vi "Value_Occurence_Analysis.vi"(3 "Average Numeric Values?":bool, 4 "Tolerance":dbl=1.0 format="%.2f", 5 "Precision (3)":string, 6 "String Array":string[](array[string])) -> (0 "Numeric Array?":bool, 1 "St Dev":string, 2 "Output String":string)   [LabVIEW 2010]
uses:
  <vilib>/Analysis/NI_AALBase.lvlib
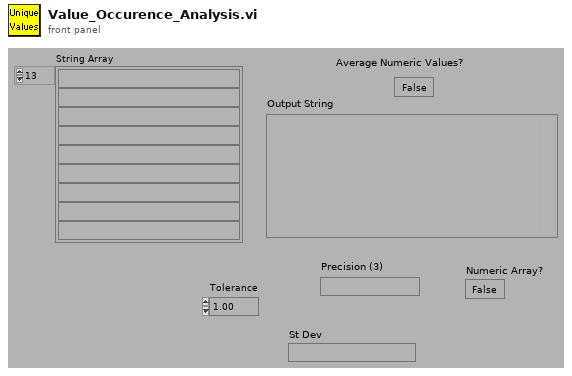
[diagram p1: front panel]
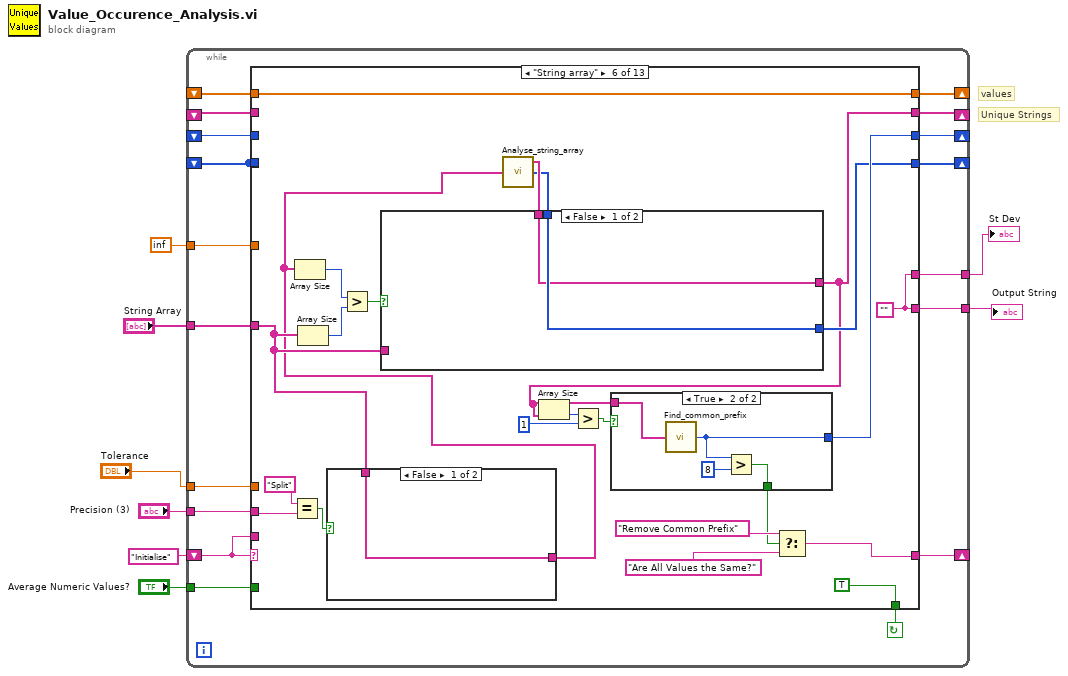
[diagram p0: block diagram]
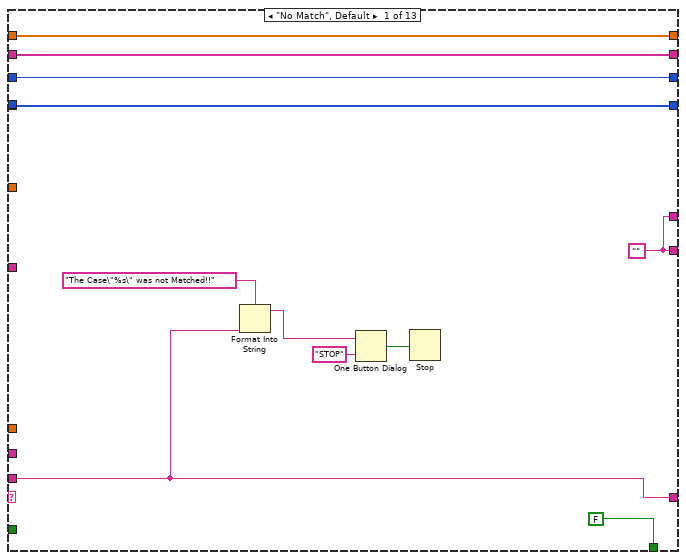
[diagram p2: hidden frame]
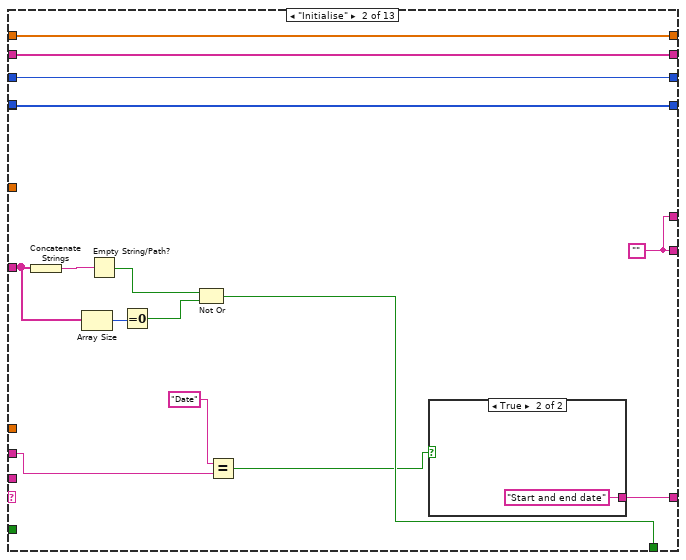
[diagram p3: hidden frame]
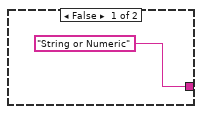
[diagram p4: hidden frame]
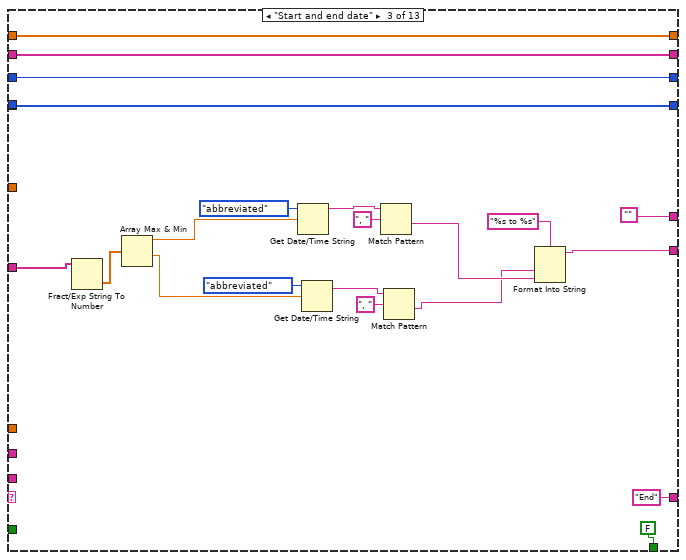
[diagram p5: hidden frame]
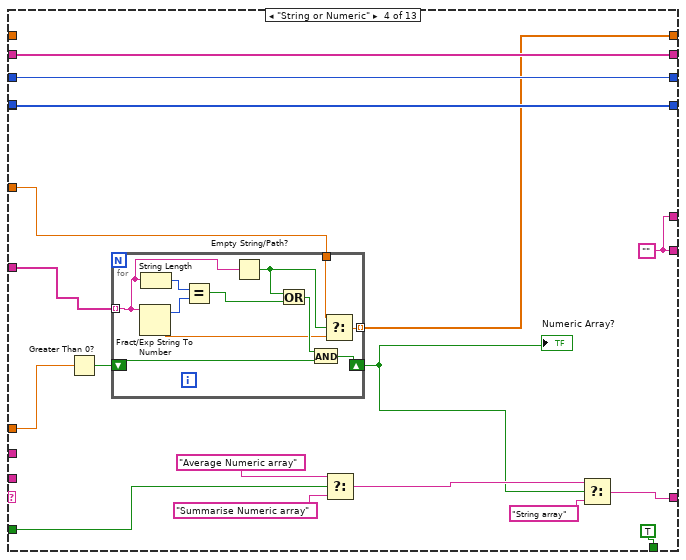
[diagram p6: hidden frame]
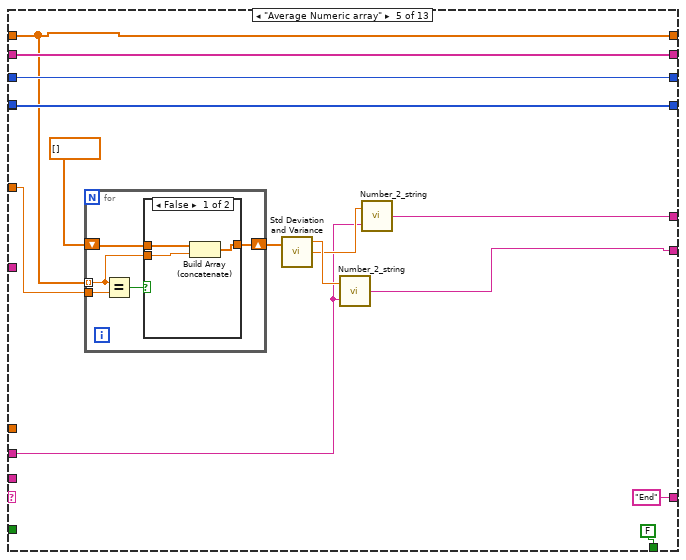
[diagram p7: hidden frame]
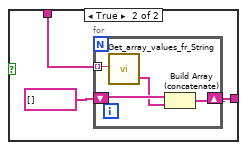
[diagram p9: hidden frame]
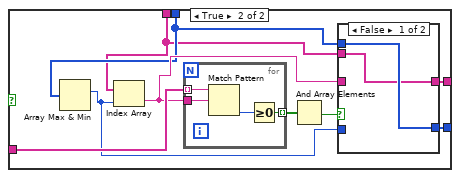
[diagram p10: hidden frame]
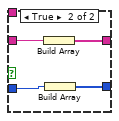
[diagram p11: hidden frame]
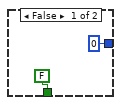
[diagram p12: hidden frame]
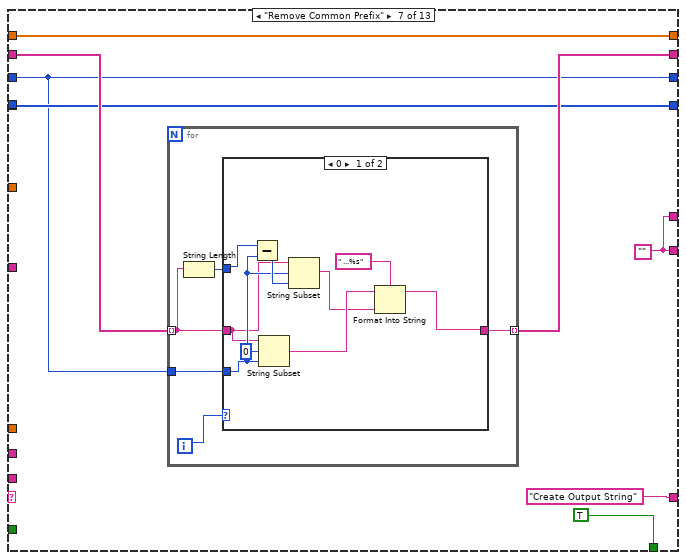
[diagram p13: hidden frame]
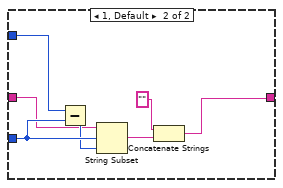
[diagram p14: hidden frame]
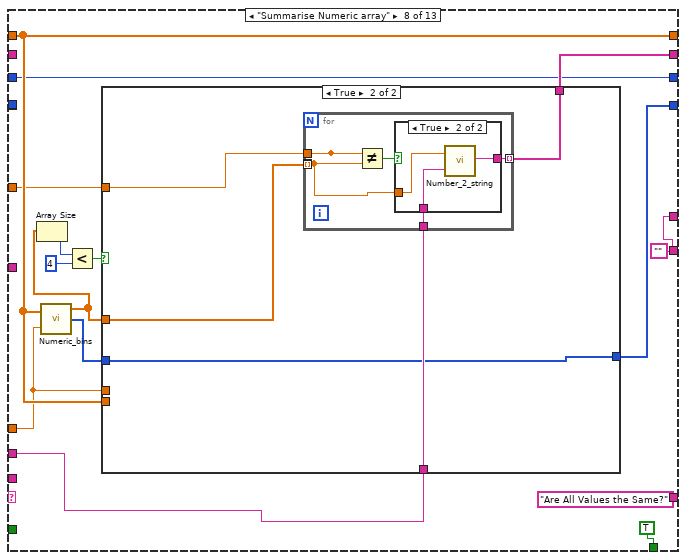
[diagram p15: hidden frame]
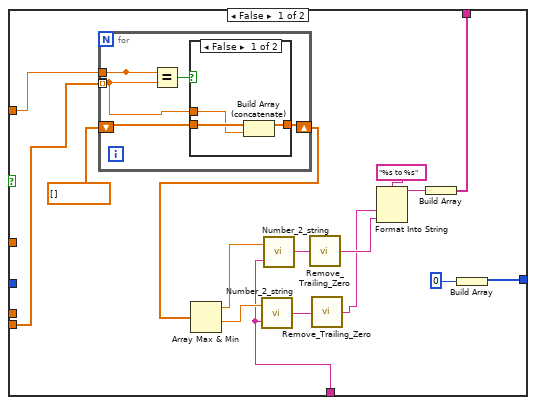
[diagram p16: hidden frame]
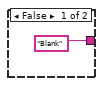
[diagram p18: hidden frame]
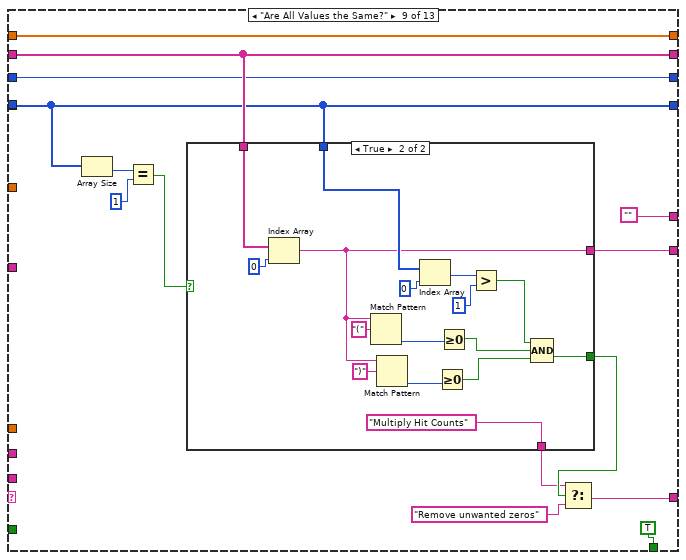
[diagram p19: hidden frame]
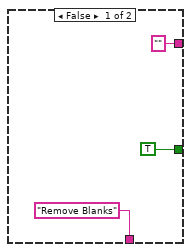
[diagram p20: hidden frame]
diagram:
  # "Unique Strings"
  # "values"
  n1 = while {
    shift-left: _ -> [w12]
    shift-right: [w13] -> _
    tunnel: [w14] -> w6
    shift-left: _ -> [w15]
    shift-right: [w16] -> _
    shift-left: _ -> [w17]
    shift-right: [w18] -> _
    tunnel: "Tolerance" -> [w19]
    shift-left: _ -> [w20]
    shift-right: [w24] -> _
    shift-left: "Initialise" -> [w21]
    shift-right: [w23] -> _
    tunnel: inf -> [w25]
    tunnel: "String Array" -> [w26]
    tunnel: "Average Numeric Values?" -> [w11]
    tunnel: "Precision (3)" -> [w10]
    tunnel: [w9] -> w2
    stop <- w22 continue-if-true
    n2 = case shown="\"String array\"" w21 {
      tunnel: w26 -> [_ w47 w62 w88 _ w135 _ _ _ _ _ _ _]
      tunnel: w25 -> [_ _ _ w76 w111 _ _ w223 _ _ _ _ _]
      tunnel: [w32 w52 w71 w77 w110 w148 w191 w225 w281 w313 w345 w378 w396] -> w24
      tunnel: [w33 w49 "End" w91 "End" w143 "Create Output String" "Are All Values the Same?" w269 "End" "Remove unwanted zeros" "Create Output String" "Initialise"] -> w23
      tunnel: [FALSE w43 FALSE TRUE FALSE TRUE TRUE TRUE TRUE FALSE TRUE TRUE FALSE] -> w22
      tunnel: w21 -> [w33 _ _ _ _ _ _ _ _ _ _ _ _]
      tunnel: w20 -> [w32 w52 w71 _ w110 w148 w191 w225 w281 w313 w345 w378 w396]
      tunnel: w19 -> [_ _ _ w86 _ _ _ w224 _ _ _ _ _]
      tunnel: [w30 w51 w73 w89 w116 w132 w187 w222 w274 w310 w342 w377 w386] -> w18
      tunnel: w17 -> [w30 w51 w73 w89 w116 _ w187 _ w274 w310 w344 w377 w386]
      tunnel: w17 -> [_ _ _ _ _ _ _ _ _ _ _ _ _]
      tunnel: [w29 w50 w75 w90 w117 w131 w189 w226 w278 w312 w343 w374 w393] -> w16
      tunnel: w15 -> [w29 w50 w75 w90 w117 _ w188 _ w278 w312 w341 w375 w393]
      tunnel: [w27 w41 w65 w78 w112 w139 w185 w214 w276 w304 w339 w373 w392] -> w14
      tunnel: [w28 w42 w74 w84 w114 w147 w186 w217 w277 w311 w340 w376 w391] -> w13
      tunnel: w12 -> [w28 w42 w74 w84 w114 _ w186 w217 w277 w311 w340 w376 w391]
      tunnel: w11 -> [_ _ _ w83 _ _ _ _ _ _ _ _ _]
      tunnel: w10 -> [_ w40 _ _ w105 w130 _ w215 _ _ _ _ _]
      tunnel: [w27 w41 "" w78 w104 w139 w185 w214 "" "" w339 w373 ""] -> w9
      frame "No Match", Default {
        w27 = ""
        n3 = Format Into String(format string="The Case\"%s\" was not Matched!!" ("Format String"), w33) -> (resulting string=w36:string)  [unwired: 2 in, 1 out]
        n4 = One Button Dialog(message=w36, button name ("OK")="STOP") -> (true=w31:bool)
        n5 = Stop(stop? (T)=w31) -> ()
      }
      frame "Initialise" {
        w41 = ""
        n6 = Concatenate Strings(w47) -> (w48:string)
        n7 = Array Size(array=w47) -> (size(s)=w45:i32)
        n8 = Empty String/Path?(string/path=w48) -> (empty?=w46:bool)
        n9 = Equal To 0?(x=w45) -> (x = 0?=w44:bool)
        n10 = Not Or(1:w44, 2:w46) -> (0:w43:bool)
        n11 = Equal?(x="Date", y=w40) -> (x = y?=w38:bool)
        n12 = case shown="True" w38 {
          tunnel: ["String or Numeric" "Start and end date"] -> w49
          frame False {
          }
          frame True {
          }
        }
      }
      frame "Start and end date" {
        n13 = Fract/Exp String To Number(string=w62) -> (number=w61:dbl[])  [unwired: 4 out]
        n14 = Array Max & Min(array=w61) -> (max value=w70:dbl, min value=w67:dbl)  [unwired: 2 out]
        n15 = Get Date/Time String(date format (0)=enum16{"short", "long", "abbreviated"}."abbreviated", seconds (now)=w70) -> (date string=w59:string)  [unwired: 2 out]
        n16 = Get Date/Time String(date format (0)=enum16{"short", "long", "abbreviated"}."abbreviated", seconds (now)=w67) -> (date string=w57:string)  [unwired: 2 out]
        n17 = Match Pattern(string=w59, regular expression=", ") -> (after substring=w56:string)  [unwired: 4 out]
        n18 = Match Pattern(string=w57, regular expression=", ") -> (after substring=w55:string)  [unwired: 4 out]
        n19 = Format Into String(format string="%s to %s", w55, w56) -> (resulting string=w65:string)  [unwired: 2 in, 1 out]
      }
      frame "String or Numeric" {
        w78 = ""
        n20 = Greater Than 0?(x=w86) -> (x > 0?=w85:bool)
        n21 = for {
          tunnel: w88 -> [w94] mode=indexing
          shift-right: [w101] -> w79
          shift-left: w85 -> [w102]
          tunnel: [w98] -> w77 mode=indexing
          tunnel: w76 -> [w99]
          n22 = Fract/Exp String To Number(string=w94) -> (offset past number=w96:i32, number=w97:dbl)  [unwired: 3 out]
          n23 = String Length(string=w94) -> (length=w95:i32)
          n24 = Equal?(x=w95, y=w96) -> (x = y?=w93:bool)
          n25 = Empty String/Path?(string/path=w94) -> (empty?=w100:bool)
          n26 = Or(x=w100, y=w93) -> (x .or. y?=w103:bool)
          n27 = And(x=w103, y=w102) -> (x .and. y?=w101:bool)
          n28 = Select(t=w99, s=w100, f=w97) -> (s? t:f=w98:dbl)
        }
        "Numeric Array?" <- w79
        n29 = Select(t="Average Numeric array", s=w83, f="Summarise Numeric array") -> (s? t:f=w80:string)
        n30 = Select(t=w80, s=w79, f="String array") -> (s? t:f=w91:string)
      }
      frame "Average Numeric array" {
        n31 = for {
          shift-right: [w118] -> w108
          shift-left: dbl[] [] -> [w120]
          tunnel: w111 -> [w122]
          tunnel: w110 -> [w119] mode=indexing
          n32 = Equal?(x=w119, y=w122) -> (x = y?=w121:bool)
          n33 = case shown="False" w121 {
            tunnel: w120 -> [w125 w126]
            tunnel: w119 -> [w124 _]
            tunnel: [w123 w126] -> w118
            frame False {
              n34 = Build Array (concatenate)(w125, w124) -> (w123:dbl[])
            }
            frame True {
            }
          }
        }
        n35 = call <vilib>:"Std Deviation and Variance.vi"("X"=w108) -> ("mean"=w107:dbl, "standard deviation"=w106:dbl)  [unwired: 1 in, 1 out]
        n36 = call "Number_2_string.vi"("precision"=w105, "number"=w107) -> ("String"=w112:string)
        n37 = call "Number_2_string.vi"("precision"=w105, "number"=w106) -> ("String"=w104:string)
      }
      frame "String array" {
        w139 = ""
        n38 = Equal?(x="Split", y=w130) -> (x = y?=w127:bool)
        n39 = Array Size(array=w135) -> (size(s)=w137:i32)
        n40 = case shown="False" w127 {
          tunnel: [w150 w152] -> w128
          tunnel: w135 -> [w150 w151]
          frame False {
          }
          frame True {
            n41 = for {
              tunnel: w151 -> [w157] mode=indexing
              shift-right: [w155] -> w152
              shift-left: string[] [] -> [w156]
              n42 = call "Get_array_values_fr_String.vi"("String Value"=w157) -> ("String array"=w154:string[])  [unwired: 1 out]
              n43 = Build Array (concatenate)(w156, w154) -> (w155:string[])
            }
          }
        }
        n44 = Array Size(array=w128) -> (size(s)=w138:i32)
        n45 = Greater?(x=w138, y=w137) -> (0:w136:bool)
        n46 = call "Analyse_string_array.vi"("String array"=w128) -> ("Unique strings"=w134:string[], "Frequency"=w133:i32[])  [unwired: 1 out]
        n47 = case shown="False" w136 {
          tunnel: w133 -> [w159 w161]
          tunnel: w134 -> [w158 w160]
          tunnel: w135 -> [_ w168]
          tunnel: [w158 w163] -> w131
          tunnel: [w159 w162] -> w132
          frame False {
          }
          frame True {
            n48 = Array Max & Min(array=w161) -> (max index (indices)=w165:i32)  [unwired: 3 out]
            n49 = Index Array(array=w160, index=w165) -> (element=w164:string)
            n50 = for {
              tunnel: w164 -> [w178]
              tunnel: w168 -> [w177] mode=indexing
              tunnel: [w175] -> w167 mode=indexing
              n51 = Match Pattern(string=w177, regular expression=w178) -> (offset past match=w176:i32)  [unwired: 4 out]
              n52 = Greater Or Equal To 0?(x=w176) -> (x >= 0?=w175:bool)
            }
            n53 = And Array Elements(Boolean array=w167) -> (logical AND=w166:bool)
            n54 = case shown="False" w166 {
              tunnel: w165 -> [_ w174]
              tunnel: w164 -> [_ w173]
              tunnel: [w169 w172] -> w163
              tunnel: [w170 w171] -> w162
              tunnel: w161 -> [w170 _]
              tunnel: w160 -> [w169 _]
              frame False {
              }
              frame True {
                n55 = Build Array(w173) -> (w172:string[])
                n56 = Build Array(w174) -> (w171:i32[])
              }
            }
          }
        }
        n57 = Array Size(array=w131) -> (size(s)=w142:i32)
        n58 = Greater?(x=w142, y=1) -> (0:w141:bool)
        n59 = case shown="True" w141 {
          tunnel: w131 -> [_ w184]
          tunnel: [0 ("Common Characters") w183] -> w147
          tunnel: [FALSE w182] -> w144
          frame False {
          }
          frame True {
            n60 = call "Find_common_prefix.vi"("Input Array"=w184) -> ("Common Characters"=w183:i32)
            n61 = Greater?(x=w183, y=8) -> (0:w182:bool)
          }
        }
        n62 = Select(t="Remove Common Prefix", s=w144, f="Are All Values the Same?") -> (s? t:f=w143:string)
      }
      frame "Remove Common Prefix" {
        w185 = ""
        n63 = for {
          tunnel: [w196] -> w189 mode=indexing
          tunnel: w188 -> [w194] mode=indexing
          tunnel: w186 -> [w195]
          i -> [w197]
          n64 = String Length(string=w194) -> (length=w193:i32)
          n65 = case shown="0" w197 {
            tunnel: [w198 w210] -> w196
            tunnel: w194 -> [w202 w211]
            tunnel: w195 -> [w203 w213]
            tunnel: w193 -> [w204 w207]
            frame 0 {
              n66 = Subtract(x=w204, y=w203) -> (x-y=w205:i32)
              n67 = String Subset(string=w202, offset (0)=0, length (rest)=w203) -> (substring=w201:string)
              n68 = String Subset(string=w202, offset (0)=w203, length (rest)=w205) -> (substring=w200:string)
              n69 = Format Into String(format string=" ...%s" ("Format String"), initial string=w201, w200) -> (resulting string=w198:string)  [unwired: 1 in, 1 out]
            }
            frame 1, Default {
              n70 = Subtract(x=w207, y=w213) -> (x-y=w212:i32)
              n71 = String Subset(string=w211, offset (0)=w213, length (rest)=w212) -> (substring=w209:string)
              n72 = Concatenate Strings("" ("Substring"), w209) -> (w210:string)
            }
          }
        }
      }
      frame "Summarise Numeric array" {
        w214 = ""
        n73 = call "Numeric_bins.vi"("Values"=w225, "Tolerance"=w224) -> ("Bin Centres"=w221:dbl[], "No of points in bins"=w216:i32[])  [unwired: 1 out]
        n74 = Array Size(array=w221) -> (size(s)=w220:i32)
        n75 = Less?(x=w220, y=4) -> (x < y?=w218:bool)
        n76 = case shown="True" w218 {
          tunnel: [w242 w258] -> w226
          tunnel: w225 -> [w236 _]
          tunnel: w224 -> [_ _]
          tunnel: w221 -> [_ w255]
          tunnel: w223 -> [w233 w256]
          tunnel: [w241 w254] -> w222
          tunnel: w215 -> [w237 w257]
          tunnel: w216 -> [_ w254]
          frame False {
            n77 = for {
              tunnel: [w245] -> _ mode=indexing
              tunnel: [w248] -> _ mode=indexing
              tunnel: w236 -> [w245] mode=indexing
              tunnel: w233 -> [w248]
              shift-right: [w246] -> w234
              shift-left: dbl[] [] -> [w247]
              n78 = Equal?(x=w248, y=w245) -> (x = y?=w249:bool)
              n79 = case shown="False" w249 {
                tunnel: w245 -> [w251 _]
                tunnel: w247 -> [w252 w253]
                tunnel: [w250 w253] -> w246
                frame False {
                  n80 = Build Array (concatenate)(w252, w251) -> (w250:dbl[])
                }
                frame True {
                }
              }
            }
            n81 = Array Max & Min(array=w234) -> (max value=w239:dbl, min value=w238:dbl)  [unwired: 2 out]
            n82 = call "Number_2_string.vi"("precision"=w237, "number"=w238) -> ("String"=w232:string)
            n83 = call "Number_2_string.vi"("precision"=w237, "number"=w239) -> ("String"=w231:string)
            n84 = call "Remove_Trailing_Zero.vi"("f"=w231) -> ("f 2"=w230:string)
            n85 = call "Remove_Trailing_Zero.vi"("f"=w232) -> ("f 2"=w229:string)
            n86 = Format Into String(format string="%s to %s" ("Format String"), w229, w230) -> (resulting string=w243:string)  [unwired: 2 in, 1 out]
            n87 = Build Array(w243) -> (w242:string[])
            n88 = Build Array(0) -> (w241:i32[])
          }
          frame True {
            n89 = for {
              tunnel: [w259] -> _ mode=indexing
              tunnel: [w261] -> _ mode=indexing
              tunnel: [w262] -> w258 mode=indexing
              tunnel: w255 -> [w259] mode=indexing
              tunnel: w256 -> [w261]
              tunnel: w257 -> [w260]
              n90 = Not Equal?(x=w261, y=w259) -> (x != y?=w263:bool)
              n91 = case shown="True" w263 {
                tunnel: ["Blank" ("f") w267] -> w262
                tunnel: w259 -> [_ w266]
                tunnel: w260 -> [_ w265]
                frame False {
                }
                frame True {
                  n92 = call "Number_2_string.vi"("precision"=w265, "number"=w266) -> ("String"=w267:string)
                }
              }
            }
          }
        }
      }
      frame "Are All Values the Same?" {
        n93 = Array Size(array=w274) -> (size(s)=w279:i32)
        n94 = Equal?(x=w279, y=1) -> (x = y?=w275:bool)
        n95 = case shown="True" w275 {
          tunnel: w278 -> [_ w299]
          tunnel: ["" ("f") w285] -> w276
          tunnel: [TRUE w292] -> w271
          tunnel: w274 -> [_ w290]
          tunnel: ["Remove Blanks" "Multiply Hit Counts"] -> w270
          frame False {
          }
          frame True {
            n96 = Index Array(array=w299, index=0 ("Index")) -> (element=w285:string)
            n97 = Match Pattern(string=w285, regular expression="(") -> (offset past match=w296:i32)  [unwired: 4 out]
            n98 = Match Pattern(string=w285, regular expression=")") -> (offset past match=w295:i32)  [unwired: 4 out]
            n99 = Index Array(array=w290, index=0 ("Index")) -> (element=w289:i32)
            n100 = Greater Or Equal To 0?(x=w295) -> (x >= 0?=w294:bool)
            n101 = Greater Or Equal To 0?(x=w296) -> (x >= 0?=w293:bool)
            n102 = Greater?(x=w289, y=1) -> (0:w287:bool)
            n103 = Compound Arithmetic op=AND(w287, w293, w294) -> (w292:bool)
          }
        }
        n104 = Select(t=w270, s=w271, f="Remove unwanted zeros") -> (s? t:f=w269:string)
      }
      frame "Multiply Hit Counts" {
        n105 = Index Array(array=w312, index=0 ("Index")) -> (element=w307:string)
        n106 = Index Array(array=w310, index=0 ("Index")) -> (element=w306:i32)
        n107 = while {
          shift-right: [w328] -> _
          shift-left: w307 -> [w330]
          shift-right: [w319] -> w304
          shift-left: "" -> [w318]
          tunnel: w306 -> [w322]
          stop <- w326 continue-if-true
          n108 = Match Pattern(string=w330, regular expression="(") -> (before substring=w325:string, match substring=w324:string, after substring=w331:string)  [unwired: 2 out]
          n109 = Match Pattern(string=w331, regular expression=")") -> (before substring=w314:string, match substring=w320:string, after substring=w328:string)  [unwired: 2 out]
          n110 = Decimal String To Number(string=w314) -> (offset past number=w316:i32, number=w323:i32)  [unwired: 2 out]
          n111 = String Length(string=w314) -> (length=w317:i32)
          n112 = Match Pattern(string=w328, regular expression="(") -> (offset past match=w327:i32)  [unwired: 4 out]
          n113 = Equal?(x=w316, y=w317) -> (x = y?=w315:bool)
          n114 = case shown="True" w315 {
            tunnel: w323 -> [_ w338]
            tunnel: w322 -> [_ w337]
            tunnel: [w334 w335] -> w321
            tunnel: w314 -> [w334 _]
            frame False {
            }
            frame True {
              n115 = Multiply(x=w337, y=w338) -> (x*y=w336:i32)
              n116 = Number To Decimal String(number=w336) -> (decimal integer string=w335:string)  [unwired: 1 out]
            }
          }
          n117 = Greater Or Equal To 0?(x=w327) -> (x >= 0?=w326:bool)
          n118 = Concatenate Strings(w318, w325, w324, w321, w320) -> (w319:string)
        }
      }
      frame "Remove Blanks" {
        w339 = ""
        n119 = Empty String/Path?(string/path=w341) -> (empty?=w347:bool[])
        n120 = Or Array Elements(Boolean array=w347) -> (logical OR=w346:bool)
        n121 = case shown="True" w346 {
          tunnel: w341 -> [w350 w352]
          tunnel: w344 -> [w351 w357]
          tunnel: [w350 w354] -> w343
          tunnel: [w351 w353] -> w342
          frame False {
          }
          frame True {
            n122 = for {
              shift-right: [w361] -> w354
              shift-left: string[] [] -> [w362]
              shift-right: [w360] -> w353
              shift-left: i32[] [] -> [w363]
              tunnel: w352 -> [w358] mode=indexing
              tunnel: w357 -> [w359] mode=indexing
              n123 = Empty String/Path?(string/path=w358) -> (empty?=w364:bool)
              n124 = case shown="False" w364 {
                tunnel: w363 -> [w370 w371]
                tunnel: w362 -> [w369 w372]
                tunnel: [w368 w372] -> w361
                tunnel: [w367 w371] -> w360
                tunnel: w358 -> [w366 _]
                tunnel: w359 -> [w365 _]
                frame False {
                  n125 = Build Array (concatenate)(w369, w366) -> (w368:string[])
                  n126 = Build Array (concatenate)(w370, w365) -> (w367:i32[])
                }
                frame True {
                }
              }
            }
          }
        }
      }
      frame "Remove unwanted zeros" {
        w373 = ""
        n127 = for {
          tunnel: w375 -> [w381] mode=indexing
          tunnel: [w382] -> w374 mode=indexing
          n128 = call "Remove_Trailing_Zero.vi"("f"=w381) -> ("f 2"=w382:string)
        }
      }
      frame "Create Output String" {
        n129 = Array Size(array=w386) -> (size(s)=w385:i32)
        n130 = Equal?(x=w386, y=1) -> (x = y?=w389:bool[])
        n131 = Equal?(x=w385, y=1) -> (x = y?=w383:bool)
        n132 = And Array Elements(Boolean array=w389) -> (logical AND=w388:bool)
        n133 = case shown="True" w383 {
          tunnel: w393 -> [w405 w423]
          tunnel: [w399 w421] -> w392
          tunnel: w388 -> [w398 _]
          tunnel: w386 -> [w397 _]
          frame False {
            n134 = for {
              shift-right: [w410] -> w403
              shift-left: "" -> [w411]
              tunnel: w405 -> [w409] mode=indexing
              tunnel: w397 -> [w408] mode=indexing
              tunnel: w398 -> [w407]
              n135 = case shown="False" w407 {
                tunnel: w411 -> [w416 w420]
                tunnel: [w415 w419] -> w410
                tunnel: w409 -> [w414 w418]
                tunnel: w408 -> [w413 _]
                frame False {
                  n136 = Format Into String(format string="%s (%d);  " ("Format String"), initial string=w416, w414, w413) -> (resulting string=w415:string)  [unwired: 1 in, 1 out]
                }
                frame True {
                  n137 = Format Into String(format string="%s;  " ("Format String"), initial string=w420, w418) -> (resulting string=w419:string)  [unwired: 1 in, 1 out]
                }
              }
            }
            n138 = String Length(string=w403) -> (length=w401:i32)
            n139 = Subtract(x=w401, y=2) -> (x-y=w400:i32)
            n140 = String Subset(string=w403, offset (0)=0, length (rest)=w400) -> (substring=w399:string)
          }
          frame True {
            n141 = Index Array(array=w423, index=0) -> (element=w421:string)
          }
        }
      }
    }
  }
  "Output String" <- w6
  "St Dev" <- w2
